vi "Quad Octet to IP.vi"(8 "Octet 4":u8, 9 "Octet 3":u8, 10 "Octet 2":u8, 11 "Octet 1":u8) -> (3 "U32 IP":u32)   [LabVIEW 2020]
panel:
  # "."
  # "."
  # "."
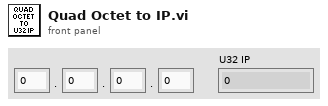
[diagram p1: front panel]
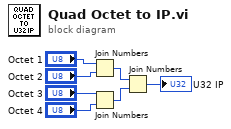
[diagram p0: block diagram]
diagram:
  n1 = Join Numbers(hi="Octet 1", lo="Octet 2") -> ((hi.lo)=w3:u16)
  n2 = Join Numbers(hi="Octet 3", lo="Octet 4") -> ((hi.lo)=w2:u16)
  n3 = Join Numbers(hi=w3, lo=w2) -> ((hi.lo)=→"U32 IP":u32)
